vi "Renishaw-XL80_ClearErrors.vi"(8 "error in (no error)":errorcluster, 11 "Renishaw-XL80 in":refnum<class "Renishaw-XL80.lvclass">) -> (0 "error out":errorcluster, 3 "Renishaw-XL80 out":refnum<class "Renishaw-XL80.lvclass">)   [LabVIEW 2024, in "Renishaw-XL80.lvclass"]
uses:
  Renishaw-XL80.lvclass
  Renishaw-XL80.lvclass/Renishaw-XL80.ctl
  D:/A.C.M/Example CSharp_64/bin/Debug/Interop.DX10SDKADAPTORLib.dll
  Example CSharp_64/bin/Debug/Interop.DX10SDKADAPTORLib.dll
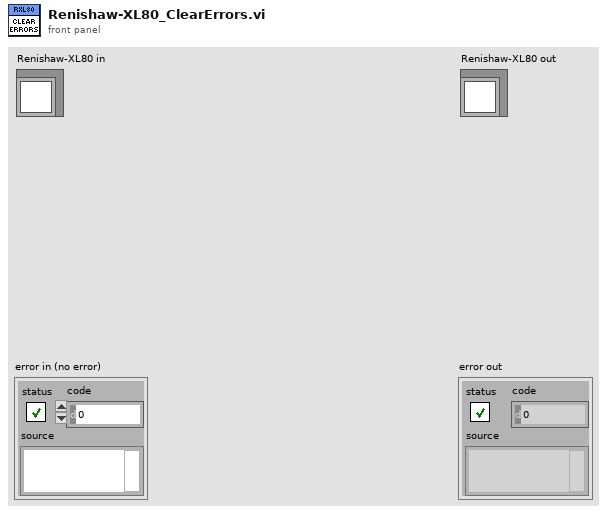
[diagram p1: front panel]
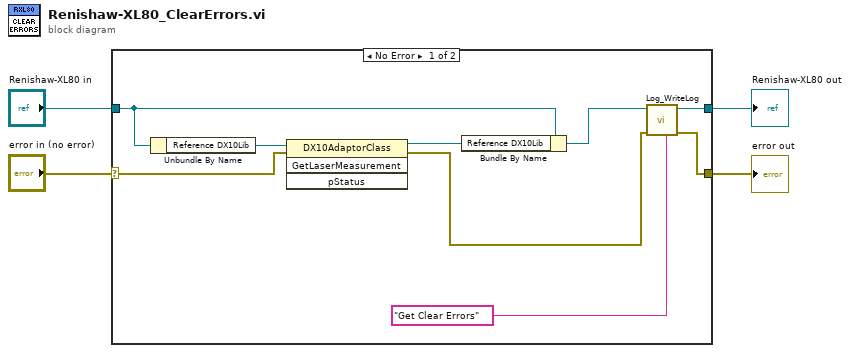
[diagram p0: block diagram]
diagram:
  n1 = case shown="No Error" "error in (no error)" {
    selector: "error in (no error)" -> [w10 w15]
    tunnel: [w8 w15] -> w1
    tunnel: [w9 w14] -> w3
    tunnel: "Renishaw-XL80 in" -> [w11 w14]
    frame No Error {
      n2 = Unbundle By Name(w11) -> ("Reference DX10Lib"=w13:refnum<k24>)
      n3 = invoke class="DX10AdaptorClass" method="GetLaserMeasurement"(reference=w13, error in=w10) -> (reference out=w12:refnum<k24>, error out=w5:errorcluster)  [unwired: 2 in, 2 out]
      n4 = Bundle By Name(cluster=w11, "Reference DX10Lib"=w12) -> (w7:refnum<class "Renishaw-XL80.lvclass">)
      n5 = call-dynamic "Log_WriteLog.vi"("Additional text"="Get Clear Errors", "error in (no error)"=w5, "Log in"=w7) -> ("error out"=w8:errorcluster, "Log out"=w9:refnum<class "Renishaw-XL80.lvclass">)  [unwired: 7 in]
    }
    frame Error {
    }
  }
  "error out" <- w1
  "Renishaw-XL80 out" <- w3
